vi "Inject Teller Metadata.vi"(4 "Priority":bool, 8 "Error in":errorcluster, 9 "Reply":bool, 10 "Msg":refnum<class "Msg.lvclass">, 11 "Actor in":refnum<class "Actor.lvclass">) -> (2 "Teller Metadata":refnum<class "Teller Metadata.lvclass">)   [LabVIEW 2025, in "jettl.lvlib" / "Actor.lvclass"]
uses:
  Actor.lvclass
  Teller Metadata/Teller Metadata.lvclass
  Msg/Msg.lvclass
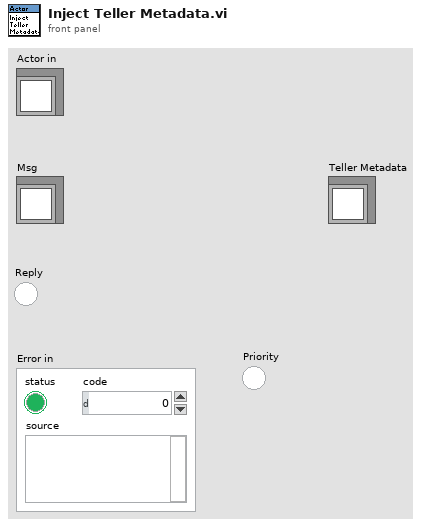
[diagram p1: front panel]
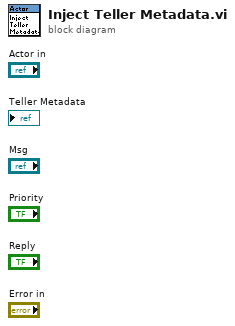
[diagram p0: block diagram]
diagram:
